vi "Set Num Periods.vi"(4 "# of periods":i32=1 min=0 max=2000 step=1, 7 "Set # Periods":bool, 8 "Error In":errorcluster caption="Error", 11 "VISA resource name":refnum<visa-resource-name>) -> (0 "Error Out":errorcluster, 3 "VISA resource name out":refnum<visa-resource-name>)   [LabVIEW 2015]
uses:
  SR400.lvlib
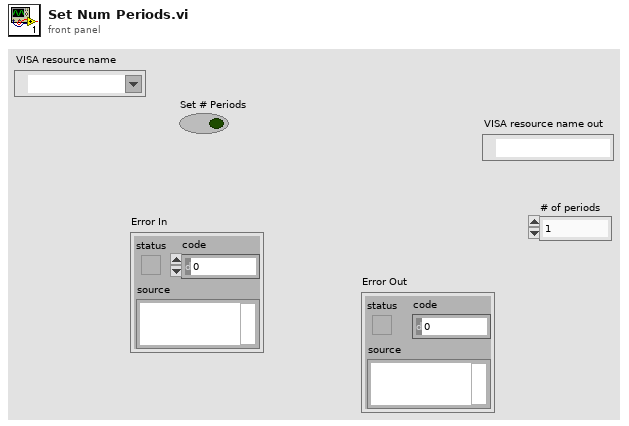
[diagram p1: front panel]
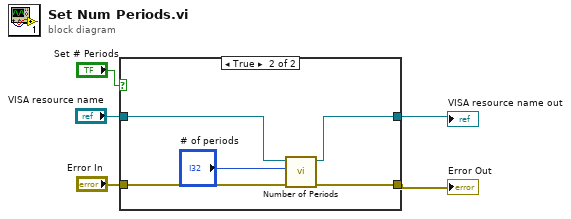
[diagram p0: block diagram]
diagram:
  n1 = case shown="True" "Set # Periods" {
    tunnel: "Error In" -> [w7 w11]
    tunnel: [w7 w8] -> w2
    tunnel: "VISA resource name" -> [w6 w12]
    tunnel: [w6 w9] -> w1
    frame False {
    }
    frame True {
      n2 = call "Number of Periods.vi"("error in (no error)"=w11, "# of periods (def: 1)"="# of periods", "VISA resource name"=w12) -> ("error out"=w8:errorcluster, "VISA resource name out"=w9:refnum<visa-resource-name>)  [unwired: 7 in]
    }
  }
  "Error Out" <- w2
  "VISA resource name out" <- w1
